vi "IS_EXE.vi"(3 "error in":errorcluster) -> (0 "error out":errorcluster, 1 "1 - EXE":bool, 2 "Application:Kind":T1(ring))   [LabVIEW 2018]
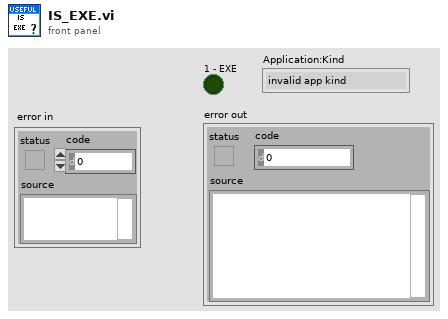
[diagram p1: front panel]
types:
  T1 = enum32{"invalid app kind", "Development System", "Run Time System", "Student Edition", "Embedded LabVIEW", "Evaluation", "Custom"}
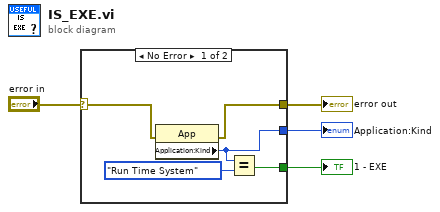
[diagram p0: block diagram]
diagram:
  n1 = case shown="No Error" "error in" {
    selector: "error in" -> [w7 w10]
    tunnel: [w8 _] -> w3
    tunnel: [w6 w10] -> w2
    tunnel: [w5 _] -> w1
    frame No Error {
      n2 = property on="Property Node" class="App"(error in=w7) -> (error out=w6:errorcluster, "Application:Kind"=w5:T1)  [unwired: 1 in, 1 out]
      n3 = Equal?(x=w5, y=T1."Run Time System") -> (x = y?=w8:bool)
    }
    frame Error {
    }
  }
  "error out" <- w2
  "1 - EXE" <- w3
  "Application:Kind" <- w1
